vi "DriveStraightCommandNavX.vi"(8 "speed":dbl=0.8, 9 "Fwd Bwd":dbl, 10 "Delay ms":u32=500, 11 "distance":dbl) -> ()   [LabVIEW 2015]
uses:
  Team Code/Robot Global Data.vi
  NavX/navX Library v2/navX Library v2.lvlib
panel:
  out "isFlat":bool
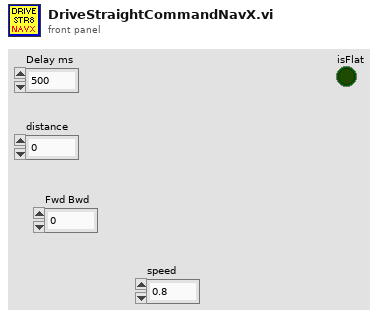
[diagram p1: front panel]
types:
  T1 = enum16{"FlatInitial", "AngleUp", "AngleDown", "FlatFinal"}
  T2 = typedef "WPI_EncoderDevRef.ctl" = cluster{"DevStatus":errorcluster, "EncoderIndex":T3, "CounterIndex":T4, "DistancePerCount":dbl, "Decoding Type":T5}
  T3 = typedef "FPGA_EncoderIdx.ctl" = enum8{"Enc 0", "Enc 1", "Enc 2", "Enc 3", "Enc 4", "Enc 5", "Enc 6", "Enc 7", "Invalid"}
  T4 = typedef "FPGA_CounterCtrSystemIndex.ctl" = enum8{"Ctr 0", "Ctr 1", "Ctr 2", "Ctr 3", "Ctr 4", "Ctr 5", "Ctr 6", "Ctr 7", "Invalid"}
  T5 = typedef "WPI_EncoderType.ctl" = enum16{"1x", "2x", "4x"}
  T6 = typedef "navX Library v2.lvlib/Z900_navX_DeviceTypeDef.ctl" = cluster{"Interface":cluster{"Protocol":T7, "Update Rate (4Hz-60Hz)":u8, "navX Open TypeDef":variant}, "Notify Packet":refnum<notifier>, "Loop VI Refnum":refnum<vi>, "Ready to Close Occurrence Refnum":refnum<k4>}
  T7 = typedef "navX Library v2.lvlib/Z900_navX_ProtocolTypeDef.ctl" = enum16{"SERIAL", "I2C", "SPI"}
  T8 = cluster{"Yaw":dbl, "Roll":dbl, "Pitch":dbl, "Heading":dbl, "Fused Heading":dbl}
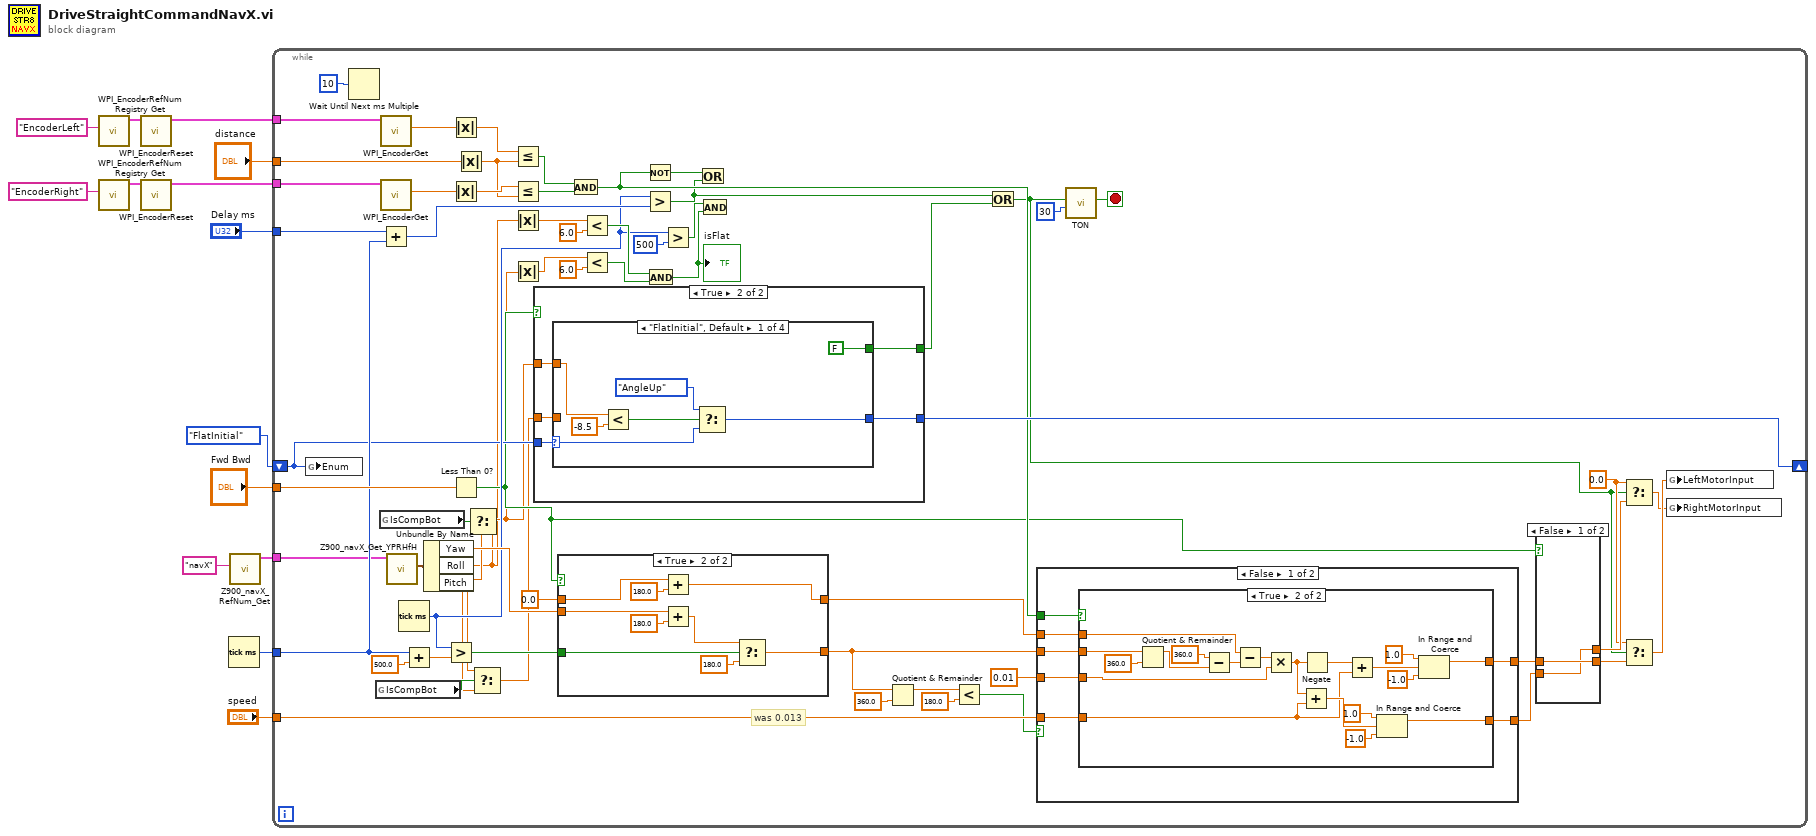
[diagram p0: block diagram]
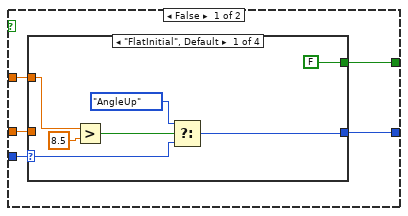
[diagram p2: hidden frame]
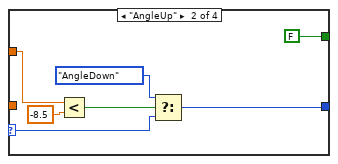
[diagram p3: hidden frame]
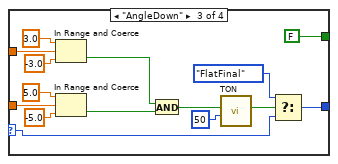
[diagram p4: hidden frame]
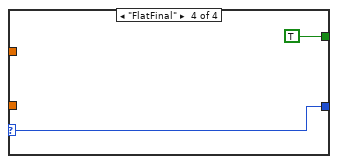
[diagram p5: hidden frame]
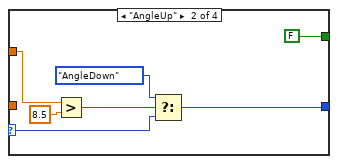
[diagram p6: hidden frame]
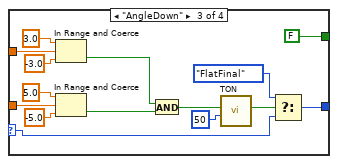
[diagram p7: hidden frame]
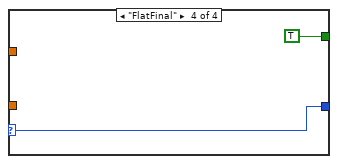
[diagram p8: hidden frame]
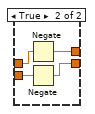
[diagram p9: hidden frame]
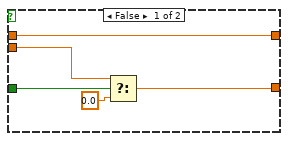
[diagram p10: hidden frame]
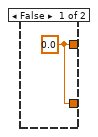
[diagram p11: hidden frame]
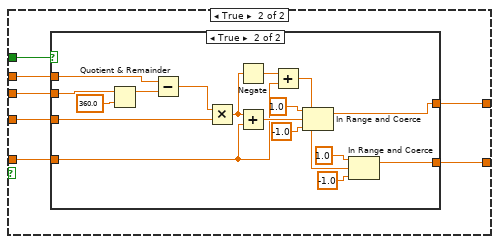
[diagram p12: hidden frame]
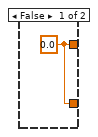
[diagram p13: hidden frame]
diagram:
  n1 = call <vilib>:"WPI_EncoderRefNum Registry Get.vi"("refnum name"="EncoderLeft") -> ("EncoderDevRef"=w13:T2)  [unwired: 9 in, 1 out]
  n2 = call <vilib>:"WPI_EncoderRefNum Registry Get.vi"("refnum name"="EncoderRight") -> ("EncoderDevRef"=w12:T2)  [unwired: 9 in, 1 out]
  n3 = call <vilib>:"WPI_EncoderReset.vi"("EncoderDevRef"=w13) -> ("EncoderDevRef"=w9:T2)  [unwired: 9 in, 1 out]
  n4 = call <vilib>:"WPI_EncoderReset.vi"("EncoderDevRef"=w12) -> ("EncoderDevRef"=w8:T2)  [unwired: 9 in, 1 out]
  n5 = Tick Count (ms)() -> (millisecond timer value=w5:u32)
  n6 = call "Z900_navX_RefNum_Get.vi"("refnum name"="navX") -> ("navX Device"=w2:T6)  [unwired: 9 in, 1 out]
  n7 = while {
    tunnel: "speed" -> [w70]
    tunnel: "distance" -> [w62]
    tunnel: w9 -> [w65]
    tunnel: w8 -> [w64]
    tunnel: "Fwd Bwd" -> [w63]
    tunnel: "Delay ms" -> [w55]
    tunnel: w5 -> [w53]
    tunnel: w2 -> [w47]
    shift-right: [w34] -> _
    shift-left: T1."FlatInitial" -> [w33]
    stop <- w25 stop-if-true
    w29 = 0.0 ("t")
    # "was 0.013"
    n8 = global write "Robot Global Data.vi" "Enum"(w33) -> ()
    n9 = Wait Until Next ms Multiple(millisecond multiple=u32 10 ("milliseconds to wait")) -> ()  [unwired: 1 out]
    n10 = global read "Robot Global Data.vi" "IsCompBot"() -> (w18:bool)
    n11 = global read "Robot Global Data.vi" "IsCompBot"() -> (w20:bool)
    n12 = call <vilib>:"WPI_EncoderGet.vi"("EncoderDevRef"=w65) -> ("Distance"=w71:dbl)  [unwired: 5 in, 5 out]
    n13 = call <vilib>:"WPI_EncoderGet.vi"("EncoderDevRef"=w64) -> ("Distance"=w74:dbl)  [unwired: 5 in, 5 out]
    n14 = Add(x=w55, y=w53) -> (x+y=w56:u32)
    n15 = call "Z900_navX_Get_YPRHfH.vi"("navX Device"=w47) -> ("YRPHfH"=w46:T8)  [unwired: 7 in, 3 out]
    n16 = Tick Count (ms)() -> (millisecond timer value=w38:u32)
    n17 = Add(x=w53, y=500.0) -> (x+y=w52:dbl)
    n18 = Unbundle By Name(w46) -> ("Yaw"=w45:dbl, "Roll"=w16:dbl, "Pitch"=w17:dbl)
    n19 = Greater?(x=w38, y=w52) -> (0:w51:bool)
    n20 = Absolute Value(x=w71) -> (abs(x)=w75:dbl)
    n21 = Absolute Value(x=w74) -> (abs(x)=w77:dbl)
    n22 = Less Than 0?(x=w63) -> (x < 0?=w21:bool)
    n23 = Absolute Value(x=w62) -> (abs(x)=w76:dbl)
    n24 = Select(t=w16, s=w20, f=w17) -> (s? t:f=w19:dbl)
    n25 = Select(t=w17, s=w18, f=w16) -> (s? t:f=w15:dbl)
    n26 = Less Or Equal?(x=w75, y=w76) -> (x <= y?=w50:bool)
    n27 = Less Or Equal?(x=w77, y=w76) -> (x <= y?=w49:bool)
    n28 = Absolute Value(x=w16) -> (abs(x)=w44:dbl)
    n29 = Absolute Value(x=w19) -> (abs(x)=w41:dbl)
    n30 = case shown="True" w21 {
      tunnel: [w79 w115] -> w34
      tunnel: w19 -> [w82 w118]
      tunnel: w33 -> [w78 w117]
      tunnel: [w80 w114] -> w23
      tunnel: w15 -> [w81 w116]
      frame False {
        n31 = case shown="\"FlatInitial\", Default" w78 {
          selector: w78 -> [w89 w96 w105 w113]
          tunnel: [w87 w94 w106 w113] -> w79
          tunnel: w82 -> [w85 w92 w111 _]
          tunnel: [FALSE FALSE FALSE TRUE] -> w80
          tunnel: w81 -> [_ _ w100 _]
          frame "FlatInitial", Default {
            n32 = Greater?(x=w85, y=8.5) -> (0:w83:bool)
            n33 = Select(t=T1."AngleUp", s=w83, f=w89) -> (s? t:f=w87:T1)
          }
          frame "AngleUp" {
            n34 = Less?(x=w92, y=-8.5) -> (x < y?=w90:bool)
            n35 = Select(t=T1."AngleDown", s=w90, f=w96) -> (s? t:f=w94:T1)
          }
          frame "AngleDown" {
            n36 = In Range and Coerce(upper limit=3.0, x=w111, lower limit=-3.0) -> (In Range?=w99:bool)  [unwired: 1 out]
            n37 = In Range and Coerce(upper limit=5.0, x=w100, lower limit=-5.0) -> (In Range?=w98:bool)  [unwired: 1 out]
            n38 = And(x=w99, y=w98) -> (x .and. y?=w97:bool)
            n39 = call "TON.vi"("Delay (ms)"=u32 50, "Input"=w97) -> ("Output"=w104:bool)  [unwired: 9 in]
            n40 = Select(t=T1."FlatFinal", s=w104, f=w105) -> (s? t:f=w106:T1)
          }
          frame "FlatFinal" {
          }
        }
      }
      frame True {
        n41 = case shown="\"FlatInitial\", Default" w117 {
          selector: w117 -> [w125 w132 w141 w149]
          tunnel: [w123 w130 w142 w149] -> w115
          tunnel: w118 -> [w121 w128 w147 _]
          tunnel: [FALSE FALSE FALSE TRUE] -> w114
          tunnel: w116 -> [_ _ w136 _]
          frame "FlatInitial", Default {
            n42 = Less?(x=w121, y=-8.5) -> (x < y?=w119:bool)
            n43 = Select(t=T1."AngleUp", s=w119, f=w125) -> (s? t:f=w123:T1)
          }
          frame "AngleUp" {
            n44 = Greater?(x=w128, y=8.5) -> (0:w126:bool)
            n45 = Select(t=T1."AngleDown", s=w126, f=w132) -> (s? t:f=w130:T1)
          }
          frame "AngleDown" {
            n46 = In Range and Coerce(upper limit=3.0, x=w147, lower limit=-3.0) -> (In Range?=w135:bool)  [unwired: 1 out]
            n47 = In Range and Coerce(upper limit=5.0, x=w136, lower limit=-5.0) -> (In Range?=w134:bool)  [unwired: 1 out]
            n48 = And(x=w135, y=w134) -> (x .and. y?=w133:bool)
            n49 = call "TON.vi"("Delay (ms)"=u32 50, "Input"=w133) -> ("Output"=w140:bool)  [unwired: 9 in]
            n50 = Select(t=T1."FlatFinal", s=w140, f=w141) -> (s? t:f=w142:T1)
          }
          frame "FlatFinal" {
          }
        }
      }
    }
    n51 = case shown="True" w21 {
      tunnel: w45 -> [w159 w169]
      tunnel: [w158 w163] -> w61
      tunnel: 0.0 ("wanted angle") -> [w160 w165]
      tunnel: [w160 w167] -> w73
      tunnel: w51 -> [w157 w162]
      frame False {
        n52 = Select(t=w159, s=w157, f=0.0) -> (s? t:f=w158:dbl)
      }
      frame True {
        n53 = Add(x=w165, y=180.0) -> (x+y=w167:dbl)
        n54 = Add(x=w169, y=180.0) -> (x+y=w164:dbl)
        n55 = Select(t=w164, s=w162, f=180.0) -> (s? t:f=w163:dbl)
      }
    }
    n56 = And(x=w50, y=w49) -> (x .and. y?=w27:bool)
    n57 = Less?(x=w44, y=6.0) -> (x < y?=w42:bool)
    n58 = Less?(x=w41, y=6.0) -> (x < y?=w39:bool)
    n59 = Not(x=w27) -> (.not. x?=w48:bool)
    n60 = Greater?(x=w38, y=w56) -> (0:w24:bool)
    n61 = And(x=w42, y=w39) -> (x .and. y?=w35:bool)
    "isFlat" <- w35
    n62 = Greater?(x=w38, y=u32 500) -> (0:w36:bool)
    n63 = Or(x=w48, y=w24) -> ()  [unwired: 1 out]
    n64 = And(x=w36, y=w35) -> ()  [unwired: 1 out]
    n65 = Quotient & Remainder(x=w61, y=360.0) -> (x-y*floor(x/y)=w66:dbl)  [unwired: 1 out]
    n66 = Less?(x=w66, y=180.0) -> (x < y?=w59:bool)
    n67 = Or(x=w24, y=w23) -> (x .or. y?=w22:bool)
    n68 = case shown="False" w59 {
      tunnel: w73 -> [w175 w203]
      tunnel: [w171 w198] -> w58
      tunnel: w70 -> [w176 w202]
      tunnel: 0.01 ("Kp Gain") -> [w173 w201]
      tunnel: w27 -> [w172 w200]
      tunnel: [w170 w197] -> w57
      tunnel: w61 -> [w174 w199]
      frame False {
        n69 = case shown="True" w172 {
          tunnel: w176 -> [_ w184]
          tunnel: w175 -> [_ w189]
          tunnel: w174 -> [_ w188]
          tunnel: w173 -> [_ w183]
          tunnel: [w177 w179] -> w170
          tunnel: [w177 w178] -> w171
          frame False {
            w177 = 0.0
          }
          frame True {
            n70 = Quotient & Remainder(x=w188, y=360.0) -> (x-y*floor(x/y)=w186:dbl)  [unwired: 1 out]
            n71 = Subtract(x=360.0, y=w186) -> (x-y=w185:dbl)
            n72 = Subtract(x=w189, y=w185) -> (x-y=w180:dbl)
            n73 = Multiply(x=w180, y=w183) -> (x*y=w181:dbl)
            n74 = Add(x=w181, y=w184) -> (x+y=w193:dbl)
            n75 = Negate(x=w181) -> (-x=w182:dbl)
            n76 = Add(x=w182, y=w184) -> (x+y=w190:dbl)
            n77 = In Range and Coerce(upper limit=1.0, x=w193, lower limit=-1.0) -> (coerced(x)=w179:dbl)  [unwired: 1 out]
            n78 = In Range and Coerce(upper limit=1.0, x=w190, lower limit=-1.0) -> (coerced(x)=w178:dbl)  [unwired: 1 out]
          }
        }
      }
      frame True {
        n79 = case shown="True" w200 {
          tunnel: w203 -> [_ w218]
          tunnel: [w204 w206] -> w198
          tunnel: w202 -> [_ w211]
          tunnel: w201 -> [_ w215]
          tunnel: [w204 w205] -> w197
          tunnel: w199 -> [_ w212]
          frame False {
            w204 = 0.0 ("output")
          }
          frame True {
            n80 = Quotient & Remainder(x=w212, y=360.0) -> (x-y*floor(x/y)=w219:dbl)  [unwired: 1 out]
            n81 = Subtract(x=w218, y=w219) -> (x-y=w207:dbl)
            n82 = Multiply(x=w207, y=w215) -> (x*y=w210:dbl)
            n83 = Negate(x=w210) -> (-x=w208:dbl)
            n84 = Add(x=w210, y=w211) -> (x+y=w216:dbl)
            n85 = Add(x=w208, y=w211) -> (x+y=w209:dbl)
            n86 = In Range and Coerce(upper limit=1.0, x=w216, lower limit=-1.0) -> (coerced(x)=w206:dbl)  [unwired: 1 out]
            n87 = In Range and Coerce(upper limit=1.0, x=w209, lower limit=-1.0) -> (coerced(x)=w205:dbl)  [unwired: 1 out]
          }
        }
      }
    }
    n88 = call "TON.vi"("Delay (ms)"=u32 30, "Input"=w22) -> ("Output"=w25:bool)  [unwired: 9 in]
    n89 = case shown="False" w21 {
      tunnel: [w151 w152] -> w32
      tunnel: [w150 w153] -> w30
      tunnel: w58 -> [w151 w155]
      tunnel: w57 -> [w150 w154]
      frame False {
      }
      frame True {
        n90 = Negate(x=w155) -> (-x=w153:dbl)
        n91 = Negate(x=w154) -> (-x=w152:dbl)
      }
    }
    n92 = Select(t=w29, s=w22, f=w30) -> (s? t:f=w28:dbl)
    n93 = Select(t=w29, s=w22, f=w32) -> (s? t:f=w31:dbl)
    n94 = global write "Robot Global Data.vi" "LeftMotorInput"(w31) -> ()
    n95 = global write "Robot Global Data.vi" "RightMotorInput"(w28) -> ()
  }
